vi "M686_Ctrl_Index.vi"(8 "NewVal":variant, 9 "OldVal":variant) -> (2 "M686 - out":T1 {"Y" format="%#_8g"; "X" format="%#_8g"}, 3 "Control out":refnum<vi>)   [LabVIEW 2014]
uses:
  Type Defs/M686.ctl
panel:
  in  "M686 - in":T1 {"Y" format="%#_8g"; "X" format="%#_8g"}
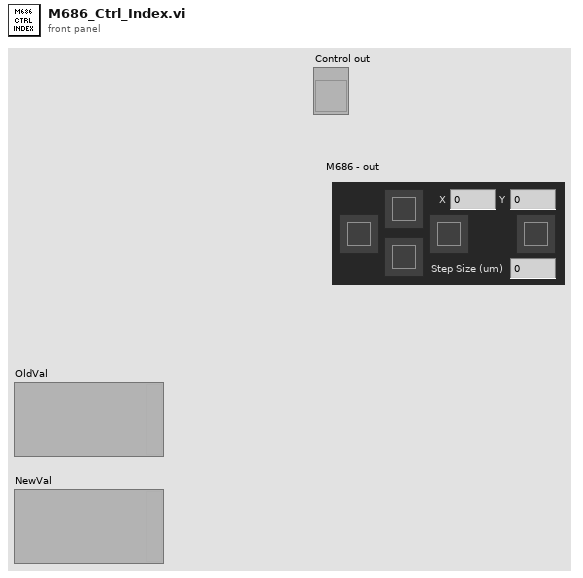
[diagram p1: front panel]
types:
  T1 = typedef "M686.ctl" = cluster{"Home Button":bool, "Left Button":bool, "Down Button":bool, "Right Button":bool, "Up Button":bool, "X":dbl, "Y":dbl, "Step Size (um)":dbl}
  T2 = cluster{"Home Button":bool, "Left Button":bool, "Down Button":bool, "Right Button":bool, "Up Button":bool, "X":bool, "Y":bool, "Step Size (um)":bool}
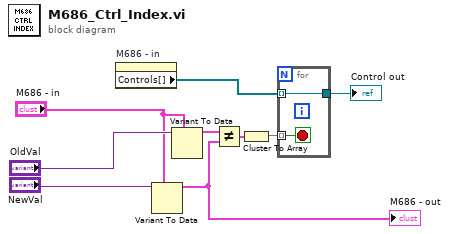
[diagram p0: block diagram]
diagram:
  n1 = property on="M686 - in" class="Clust"() -> ("Controls[]"=w1:refnum<vi>[])  [unwired: 2 in, 2 out]
  n2 = Variant To Data(type="M686 - in", Variant="NewVal") -> (data=w2:T1)  [unwired: 1 in, 1 out]
  "M686 - out" <- w2
  n3 = Variant To Data(type="M686 - in", Variant="OldVal") -> (data=w5:T1)  [unwired: 1 in, 1 out]
  n4 = Not Equal?(x=w5, y=w2) -> (x != y?=w9:T2)
  n5 = Cluster To Array(cluster=w9) -> (array=w6:bool[])
  n6 = for {
    tunnel: w6 -> [w10] mode=indexing
    tunnel: w1 -> [w11] mode=indexing
    tunnel: [w11] -> w4
    stop <- w10 stop-if-true
  }
  "Control out" <- w4
